vi "BuildLokiJson.vi"(8 "error in (no error)":errorcluster, 9 "Stream Fields Values":string[](array[string]), 10 "Stream Fields":string[](array[string]), 11 "LogRecord":refnum<class "LogRecord.lvclass">) -> (0 "error out":errorcluster, 3 "<JSON> out":string)   [LabVIEW 2019, in "hse-logger.lvlib" / "LokiJsonFormatter.lvclass"]
doc: "Example of a valid json payload to be sent to loki:\n\n{\n \"streams\": [\n {\n \"stream\": {\n \"service\": \"psu-controller\",\n \"level\": \"info\"\n },\n \"values\": [\n [\"1732457436123456789\", \"Power supply initialized\"]\n ]\n }\n ]\n}"
uses:
  LokiJsonFormatter.lvclass
  LogRecord/LogRecord.lvclass
  LogRecord/LogRecord.lvclass/LogRecord.ctl
  <vilib>/JDP Science/JSONtext/LVClass Serializer/JSONtext LVClass Serializer.lvclass
  LokiJsonFormatter.lvclass/LokiJsonFormatter.ctl
  256e9958-ef9e-487c-8968-cc0a7c9e1fb4.vi
  <vilib>/JDP Science/JSONtext/JSONtext.lvlib
  3682c22c-0fa2-43cc-a76f-2b658e9adf2b.vi
  <vilib>/Utility/error.llb/DialogType.ctl
panel:
  in  "Expected Json Structure - Just for reference":T1 caption="Expected Json Structure"
  # "Connector Pane"
  # "Locals"
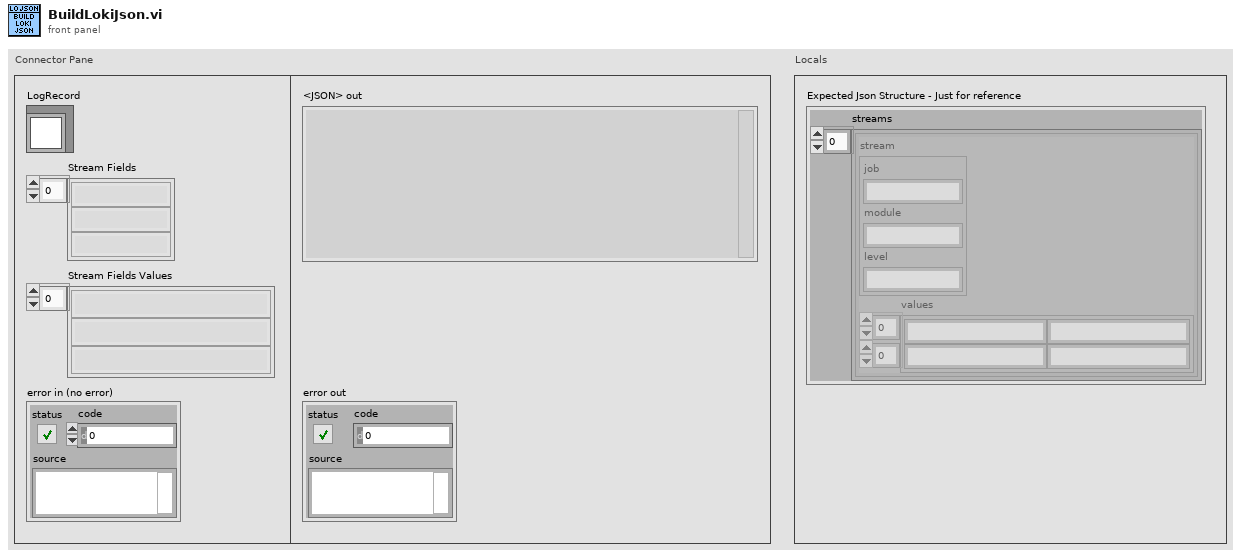
[diagram p1: front panel]
types:
  T1 = cluster{"streams":cluster{"stream":cluster{"job":string, "module":string, "level":string}, "values":string[][]}[]}
  T2 = typedef "hse-logger.lvlib/LogLevel.ctl" = enum16{"DEBUG", "INFO", "WARNING", "ERROR", "CRITICAL"}
  T3 = typedef "DialogType.ctl" = u16
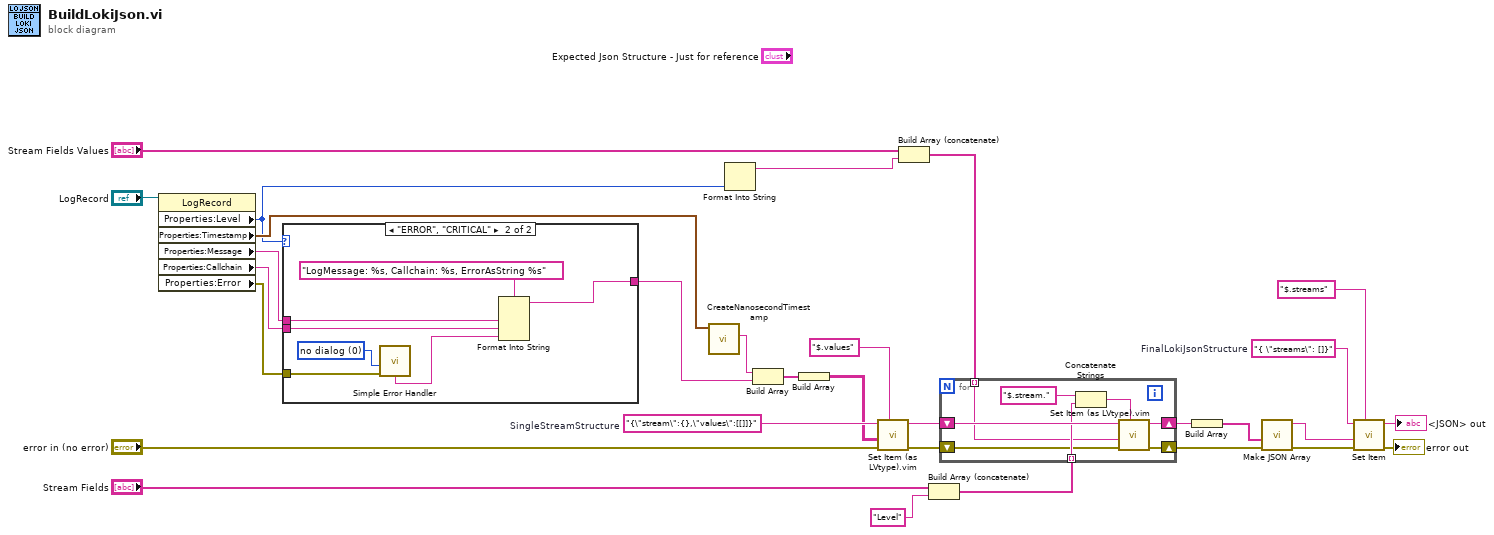
[diagram p0: block diagram]
diagram:
  w27 = "{ \"streams\": []}"  # FinalLokiJsonStructure
  w25 = "{\"stream\":{},\"values\":[[]]}"  # SingleStreamStructure
  n1 = property class="LogRecord"(reference="LogRecord") -> ("Properties:Level"=w1:T2, "Properties:Timestamp"=w2:timestamp, "Properties:Message"=w5:string, "Properties:Callchain"=w4:string, "Properties:Error"=w6:errorcluster)  [unwired: 1 in, 2 out]
  n2 = case shown="\"ERROR\", \"CRITICAL\"" w1 {
    tunnel: [w31 w32] -> w3
    tunnel: w5 -> [w31 w36]
    tunnel: w4 -> [_ w35]
    tunnel: w6 -> [_ w38]
    frame Default {
    }
    frame "ERROR", "CRITICAL" {
      w37 = T3 0 items=["no dialog", "OK message", "continue or stop message", "OK message + warnings", "continue/stop + warnings"] ("type of dialog (OK msg:1)")
      n3 = call <vilib>:"Simple Error Handler.vi"("type of dialog (OK msg:1)"=w37, "error in (no error)"=w38) -> ("message"=w34:string)  [unwired: 3 in, 4 out]
      n4 = Format Into String(format string="LogMessage: %s, Callchain: %s, ErrorAsString %s", w36, w35, w34) -> (resulting string=w32:string)  [unwired: 2 in, 1 out]
    }
  }
  n5 = call "CreateNanosecondTimestamp.vi"("current time"=w2) -> ("Timestring in RFC3339Nano"=w24:string)  [unwired: 9 in, 1 out]
  n6 = Format Into String(w1) -> (resulting string=w13:string)  [unwired: 3 in, 1 out]
  n7 = Build Array(w24, w3) -> (w23:string[])
  n8 = Build Array(w23) -> (w22:string[][])
  n9 = call "Set Item (as LVtype).vim"("$Path or Item Name"="$.values", "error in (no error)"="error in (no error)", "Anything"=w22, "JSON"=w25) -> ("error out"=w18:errorcluster, "<JSON>"=w21:string)  [unwired: 4 in, 1 out]
  n10 = Build Array (concatenate)("Stream Fields Values", w13) -> (w14:string[])
  n11 = Build Array (concatenate)("Stream Fields", "Level") -> (w16:string[])
  n12 = for {
    tunnel: w16 -> [w42] mode=indexing
    tunnel: w14 -> [w40] mode=indexing
    shift-right: [w45] -> w12
    shift-left: w21 -> [w44]
    shift-right: [w46] -> w11
    shift-left: w18 -> [w39]
    n13 = Concatenate Strings("$.stream." ("$Path or Item Name"), w42) -> (w41:string)
    n14 = call "Set Item (as LVtype).vim"("$Path or Item Name"=w41, "error in (no error)"=w39, "Anything"=w40, "JSON"=w44) -> ("error out"=w46:errorcluster, "<JSON>"=w45:string)  [unwired: 4 in, 1 out]
  }
  n15 = Build Array(w12) -> (w29:string[])
  n16 = call <vilib>:"Make JSON Array.vi"("error in (no error)"=w11, "JSON Elements"=w29) -> ("error out"=w10:errorcluster, "<JSON>"=w28:string)  [unwired: 8 in]
  n17 = call <vilib>:"Set Item.vi"("$Path or Item Name"="$.streams", "error in (no error)"=w10, "JSON to Insert"=w28, "JSON"=w27) -> ("error out"=→"error out":errorcluster, "<JSON>"=→"<JSON> out":string)  [unwired: 4 in, 1 out]
